vi "FT10_M4X Process Waveform.vi"(0 "RF Waveform In":waveform(sgl), 5 "Goertzel":cluster{"H1":dbl, "H2":dbl, "H3":dbl}={"H1"=434028.0, "H2"=1302084.0, "H3"=2170140.0}, 11 "error in":errorcluster) -> (4 "RF Waveform Out":waveform(sgl), 6 "Measurements":T1, 15 "error out":errorcluster)   [LabVIEW 2015]
doc: "Copy of \"M4X_Process Waveform.vi\" from HWT_Lillis_7854.lvproj"
uses:
  <vilib>/Waveform/WDTOps.llb/WDT Waveform Duration DBL.vi
  <vilib>/measure/matone.llb/Harmonic Distortion Analyzer 1 Chan.vi
  <vilib>/measure/matone.llb/Extract Single Tone Information 1 Chan.vi
  <vilib>/measure/madcrms.llb/Basic Averaged DC-RMS for 1 Chan.vi
  <vilib>/Waveform/WDTOps.llb/WDT Get Waveform Subset DBL.vi
  <vilib>/measure/mascope.llb/Pulse Measurements 1 chan.vi
  <vilib>/measure/NI_MAPro.lvlib
  <vilib>/Analysis/NI_AALPro.lvlib
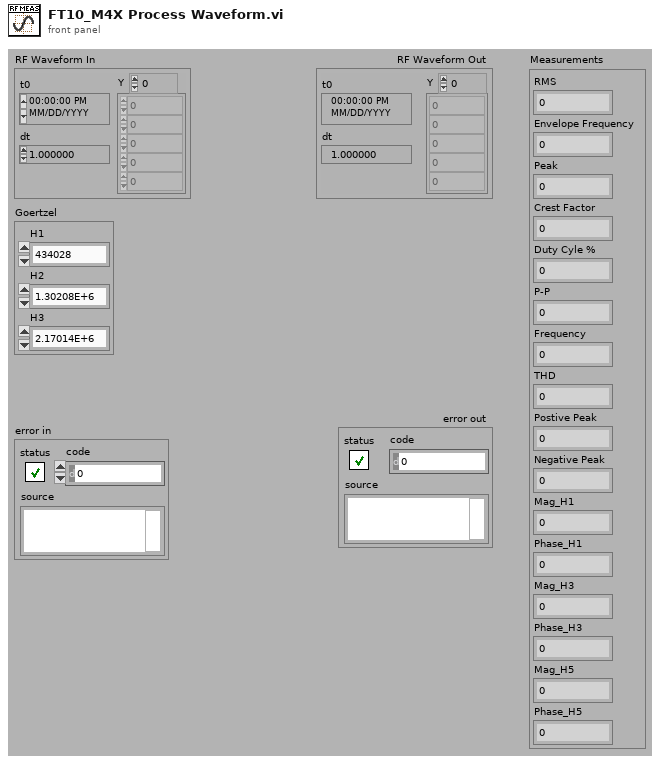
[diagram p1: front panel]
types:
  T1 = cluster{"RMS":dbl, "Envelope Frequency":dbl, "Peak":dbl, "Crest Factor":dbl, "Duty Cyle %":dbl, "P-P":dbl, "Frequency":dbl, "THD":dbl, "Postive Peak":dbl, "Negative Peak":dbl, "Mag_H1":dbl, "Phase_H1":dbl, "Mag_H3":dbl, "Phase_H3":dbl, "Mag_H5":dbl, "Phase_H5":dbl}
  T2 = cluster{"high ref level":dbl, "mid ref level":dbl, "low ref level":dbl, "ref units":u16}
  T3 = cluster{"approx freq. (optional)":dbl, "search (+/- % of Fsampl.)":dbl}
  T4 = enum32{"none", "input signal", "detected signal", "residual signal"}
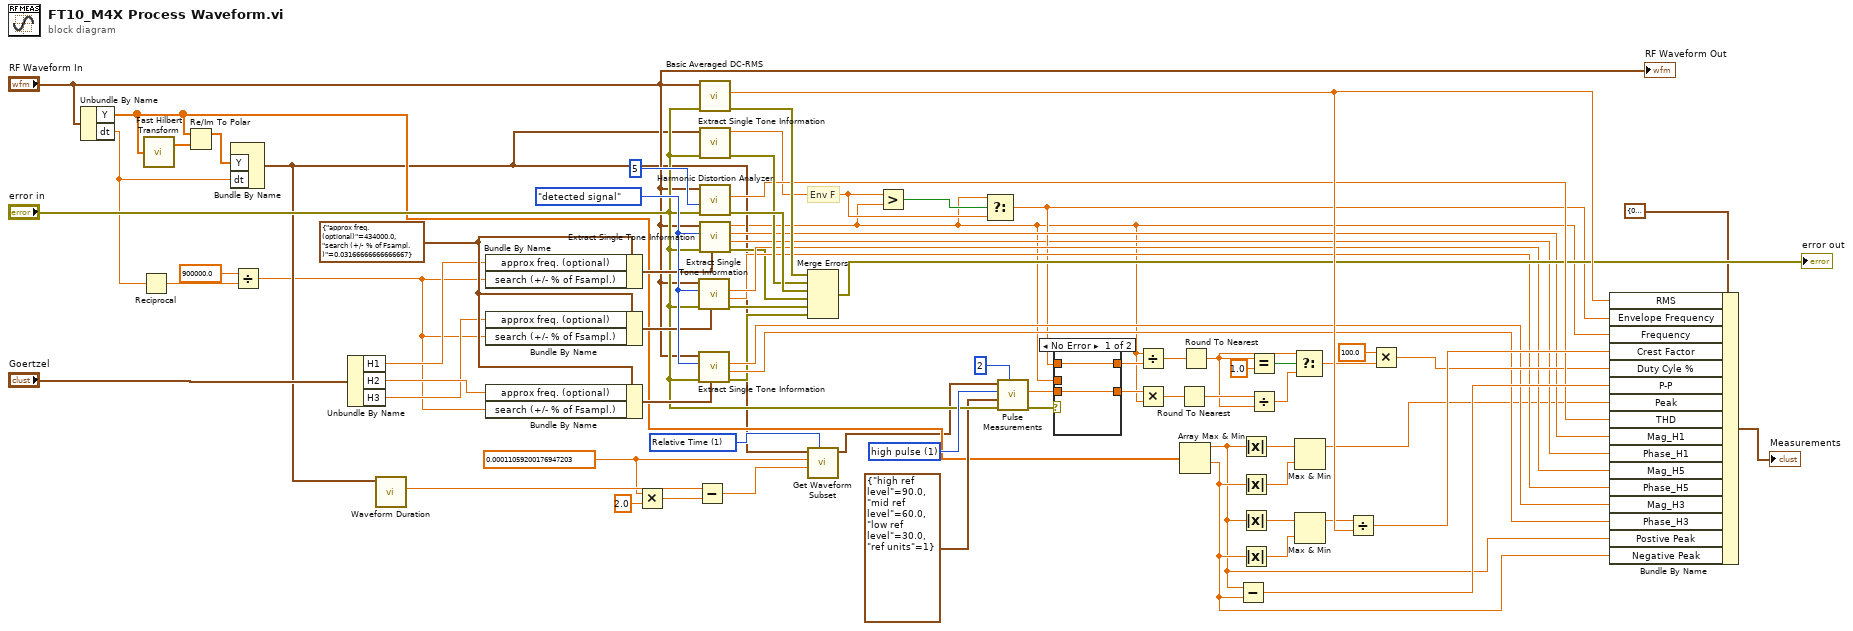
[diagram p0: block diagram]
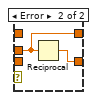
[diagram p2: hidden frame]
diagram:
  w12 = 0.00011059200176947203
  w17 = u16 1 items=["Samples", "Relative Time"] ("start/duration format")
  w41 = u16 1 items=["low pulse", "high pulse"] ("polarity (high)")
  w51 = T3 {"approx freq. (optional)"=434000.0, "search (+/- % of Fsampl.)"=0.03166666666666667} ("advanced search")
  w53 = T4."detected signal" ("export mode")
  # "Env F"
  n1 = Unbundle By Name("RF Waveform In") -> ("Y"=w18:sgl[], "dt"=w8:dbl)
  n2 = Reciprocal(x=w8) -> (1/x=w7:dbl)
  n3 = call <vilib>:"Fast Hilbert Transform.vi"("X"=w18) -> ("Hilbert{X}"=w75:dbl[])  [unwired: 1 out]
  n4 = Re/Im To Polar(2:w75, 3:w18) -> (1:w25:dbl[])  [unwired: 1 out]
  n5 = Bundle By Name("Y"=w25, "dt"=w8) -> (w10:waveform(dbl))  [unwired: 1 in]
  n6 = Divide(x=900000.0, y=w7) -> (x/y=w5:dbl)
  n7 = Unbundle By Name("Goertzel") -> ("H1"=w44:dbl, "H2"=w43:dbl, "H3"=w42:dbl)
  n8 = call-poly <vilib>:"Waveform Duration.vi"("waveform in"=w10) -> ("duration"=w16:dbl)  [unwired: 8 in, 2 out]
  n9 = Bundle By Name(cluster=w51, "approx freq. (optional)"=w44, "search (+/- % of Fsampl.)"=w5) -> (w52:T3)
  n10 = Bundle By Name(cluster=w51, "approx freq. (optional)"=w42, "search (+/- % of Fsampl.)"=w5) -> (w50:T3)
  n11 = Bundle By Name(cluster=w51, "approx freq. (optional)"=w43, "search (+/- % of Fsampl.)"=w5) -> (w49:T3)
  n12 = Multiply(x=w12, y=2.0) -> (x*y=w14:dbl)
  n13 = Subtract(x=w16, y=w14) -> (x-y=w13:dbl)
  n14 = call-poly <vilib>:"Extract Single Tone Information.vi"("advanced search"=w50, "error in (no error)"="error in", "export mode"=w53, "time signal in"="RF Waveform In") -> ("error out"=w21:errorcluster, "detected phase (deg)"=w55:dbl, "detected amplitude"=w56:dbl)  [unwired: 2 in, 3 out]
  n15 = call-poly <vilib>:"Extract Single Tone Information.vi"("advanced search"=w49, "error in (no error)"="error in", "export mode"=w53, "time signal in"="RF Waveform In") -> ("error out"=w20:errorcluster, "detected phase (deg)"=w57:dbl, "detected amplitude"=w58:dbl)  [unwired: 2 in, 3 out]
  n16 = call-poly <vilib>:"Basic Averaged DC-RMS.vi"("error in (no error)"="error in", "signal in"="RF Waveform In") -> ("error out"=w71:errorcluster, "RMS value"=w70:dbl)  [unwired: 6 in, 2 out]
  n17 = call-poly <vilib>:"Extract Single Tone Information.vi"("error in (no error)"="error in", "time signal in"=w10) -> ("error out"=w72:errorcluster, "detected frequency"=w33:dbl)  [unwired: 4 in, 4 out]
  n18 = call-poly <vilib>:"Harmonic Distortion Analyzer.vi"("error in (no error)"="error in", "highest harmonic"=5, "signal in"="RF Waveform In") -> ("error out"=w73:errorcluster, "THD"=w66:dbl)  [unwired: 3 in, 4 out]
  n19 = call-poly <vilib>:"Extract Single Tone Information.vi"("advanced search"=w52, "error in (no error)"="error in", "export mode"=w53, "time signal in"="RF Waveform In") -> ("error out"=w22:errorcluster, "detected phase (deg)"=w24:dbl, "detected amplitude"=w59:dbl, "detected frequency"=w4:dbl)  [unwired: 2 in, 2 out]
  n20 = Merge Errors(w71, w72, w73, w22, w21, w20) -> (→"error out":errorcluster)
  n21 = call-poly <vilib>:"Get Waveform Subset.vi"("start/duration format"=w17, "duration"=w13, "start samples/time"=w12, "waveform in"=w10) -> ("waveform out"=w9:waveform(dbl))  [unwired: 2 in, 3 out]
  n22 = Greater?(x=w33, y=w4) -> (0:w48:bool)
  n23 = Select(t=w4, s=w48, f=w33) -> (s? t:f=w31:dbl)
  n24 = call-poly <vilib>:"Pulse Measurements.vi"("pulse number (1)"=2, "error in (no error)"="error in", "reference levels"=T2 {"high ref level"=90.0, "mid ref level"=60.0, "low ref level"=30.0, "ref units"=1}, "polarity (high)"=w41, "signal in"=w9) -> ("error out"=w38:errorcluster, "pulse duration"=w39:dbl)  [unwired: 2 in, 3 out]
  n25 = case shown="No Error" w38 {
    tunnel: [w77 w79] -> w34
    tunnel: w39 -> [w77 _]
    tunnel: w4 -> [_ w78]
    tunnel: [w76 w78] -> w32
    tunnel: w31 -> [w76 _]
    frame No Error {
    }
    frame Error {
      n26 = Reciprocal(x=w78) -> (1/x=w79:dbl)
    }
  }
  n27 = Divide(x=w4, y=w32) -> (x/y=w36:dbl)
  n28 = Multiply(x=w34, y=w4) -> (x*y=w37:dbl)
  n29 = Round To Nearest(number=w37) -> (nearest integer value=w35:dbl)
  n30 = Array Max & Min(array=w18) -> (max value=w1:sgl, min value=w2:sgl)  [unwired: 2 out]
  n31 = Round To Nearest(number=w36) -> (nearest integer value=w28:dbl)
  n32 = Subtract(x=w1, y=w2) -> (x-y=w67:sgl)
  n33 = Absolute Value(x=w1) -> (abs(x)=w47:sgl)
  n34 = Absolute Value(x=w2) -> (abs(x)=w46:sgl)
  n35 = Absolute Value(x=w1) -> (abs(x)=w64:sgl)
  n36 = Absolute Value(x=w2) -> (abs(x)=w63:sgl)
  n37 = Equal?(x=w28, y=1.0) -> (x = y?=w29:bool)
  n38 = Divide(x=w35, y=w28) -> (x/y=w27:dbl)
  n39 = Select(t=w28, s=w29, f=w27) -> (s? t:f=w26:dbl)
  n40 = Max & Min(x=w47, y=w46) -> (max(x,y)=w3:sgl)  [unwired: 1 out]
  n41 = Max & Min(x=w64, y=w63) -> (max(x,y)=w69:sgl)  [unwired: 1 out]
  n42 = Divide(x=w69, y=w70) -> (x/y=w68:dbl)
  n43 = Multiply(x=100.0, y=w26) -> (x*y=w62:dbl)
  n44 = Bundle By Name(cluster=T1 {"RMS"=0.0, "Envelope Frequency"=0.0, "Peak"=0.0, "Crest Factor"=0.0, "Duty Cyle %"=0.0, "P-P"=0.0, "Frequency"=0.0, "THD"=0.0, "Postive Peak"=0.0, "Negative Peak"=0.0, "Mag_H1"=0.0, "Phase_H1"=0.0, "Mag_H3"=0.0, "Phase_H3"=0.0, "Mag_H5"=0.0, "Phase_H5"=0.0} ("Measurements"), "RMS"=w70, "Envelope Frequency"=w31, "Frequency"=w4, "Crest Factor"=w68, "Duty Cyle %"=w62, "P-P"=w67, "Peak"=w3, "THD"=w66, "Mag_H1"=w59, "Phase_H1"=w24, "Mag_H5"=w56, "Phase_H5"=w55, "Mag_H3"=w58, "Phase_H3"=w57, "Postive Peak"=w1, "Negative Peak"=w2) -> (→"Measurements":T1)
  "RF Waveform Out" <- "RF Waveform In"
